vi "encodeStream.vi"(8 "error in (no error)":errorcluster, 11 "tBSON_I32 in":refnum<class "tBSON_I32.lvclass">) -> (0 "error out":errorcluster, 2 "Byte Array":u8[](array[numeric]), 3 "tBSON_I32 out":refnum<class "tBSON_I32.lvclass">)   [LabVIEW 2013, in "BSON.lvlib" / "tBSON_I32.lvclass"]
uses:
  tBSON_I32.lvclass
  tBSONElement/tBSONElement.lvclass
  getValue.vi
  BSON.lvlib
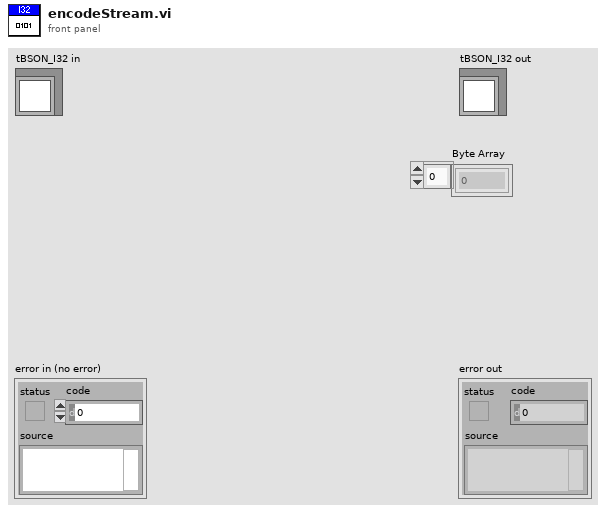
[diagram p1: front panel]
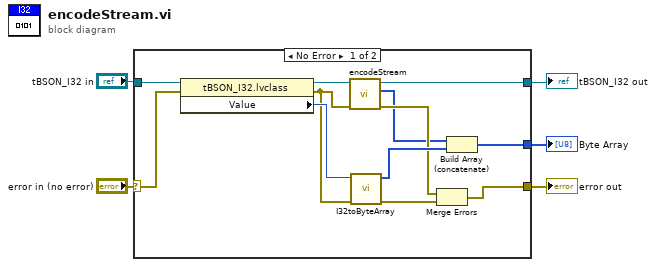
[diagram p0: block diagram]
diagram:
  n1 = case shown="No Error" "error in (no error)" {
    selector: "error in (no error)" -> [w16 w18]
    tunnel: "tBSON_I32 in" -> [w17 w19]
    tunnel: [w6 w19] -> w4
    tunnel: [w11 w18] -> w2
    tunnel: [w15 _] -> w1
    frame No Error {
      n2 = property class="tBSON_I32.lvclass"(reference=w17, error in=w16) -> (reference out=w10:refnum<class "tBSON_I32.lvclass">, error out=w9:errorcluster, "Value"=w14:i32)
      n3 = call-parent "encodeStream.vi"("error in (no error)"=w9, "tBSONElement in"=w10) -> ("error out"=w8:errorcluster, "Byte Array"=w7:u8[], "tBSONElement out"=w6:refnum<class "tBSON_I32.lvclass">)  [unwired: 7 in]
      n4 = call "I32toByteArray.vi"("error in (no error)"=w9, "I32"=w14) -> ("error out"=w12:errorcluster, "LittleEndianByteArray"=w13:u8[])  [unwired: 8 in]
      n5 = Merge Errors(w8, w12) -> (w11:errorcluster)
      n6 = Build Array (concatenate)(w7, w13) -> (w15:u8[])
    }
    frame Error {
    }
  }
  "error out" <- w2
  "tBSON_I32 out" <- w4
  "Byte Array" <- w1
